vi "FindStartEndPointsRRT.vi"(8 "Goal":dbl[](array[numeric]), 9 "Initial State":dbl[](array[numeric]), 10 "Collision Points":dbl[][](array[numeric])) -> (1 "End Point RRT":dbl[](array[numeric]), 2 "Start Point RRT":dbl[](array[numeric]))   [LabVIEW 2017]
uses:
  <vilib>/Analysis/_algsub.llb/Real Vector Norm.vi
  <vilib>/Analysis/NI_AALPro.lvlib
panel:
  in  "tamanho minimo":dbl=200.0 format="%#_13g"
  out "Start Point RRT \na ser validado":dbl[](array[numeric])
  out "End Point RRT\na ser validado":dbl[](array[numeric])
  in  "threshold":dbl=400.0 format="%#_13g"
  out "Nearest Collision Point":dbl[](array[numeric])
  out "Furthest Collision Point":dbl[](array[numeric])
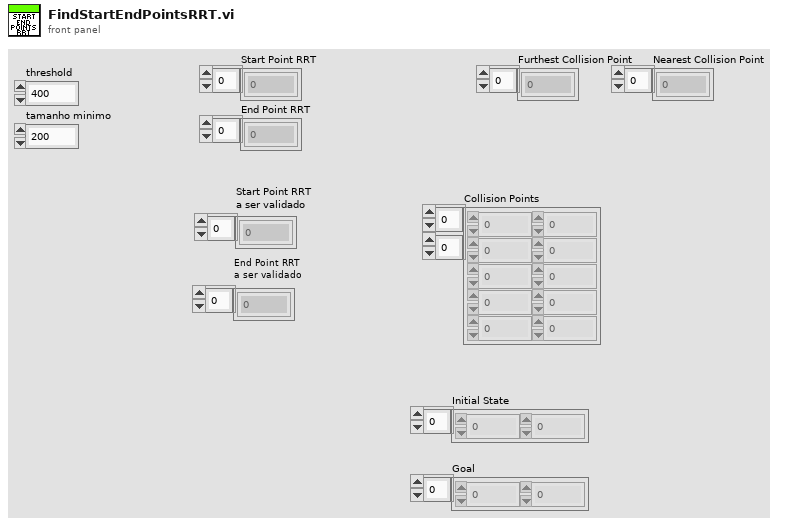
[diagram p1: front panel]
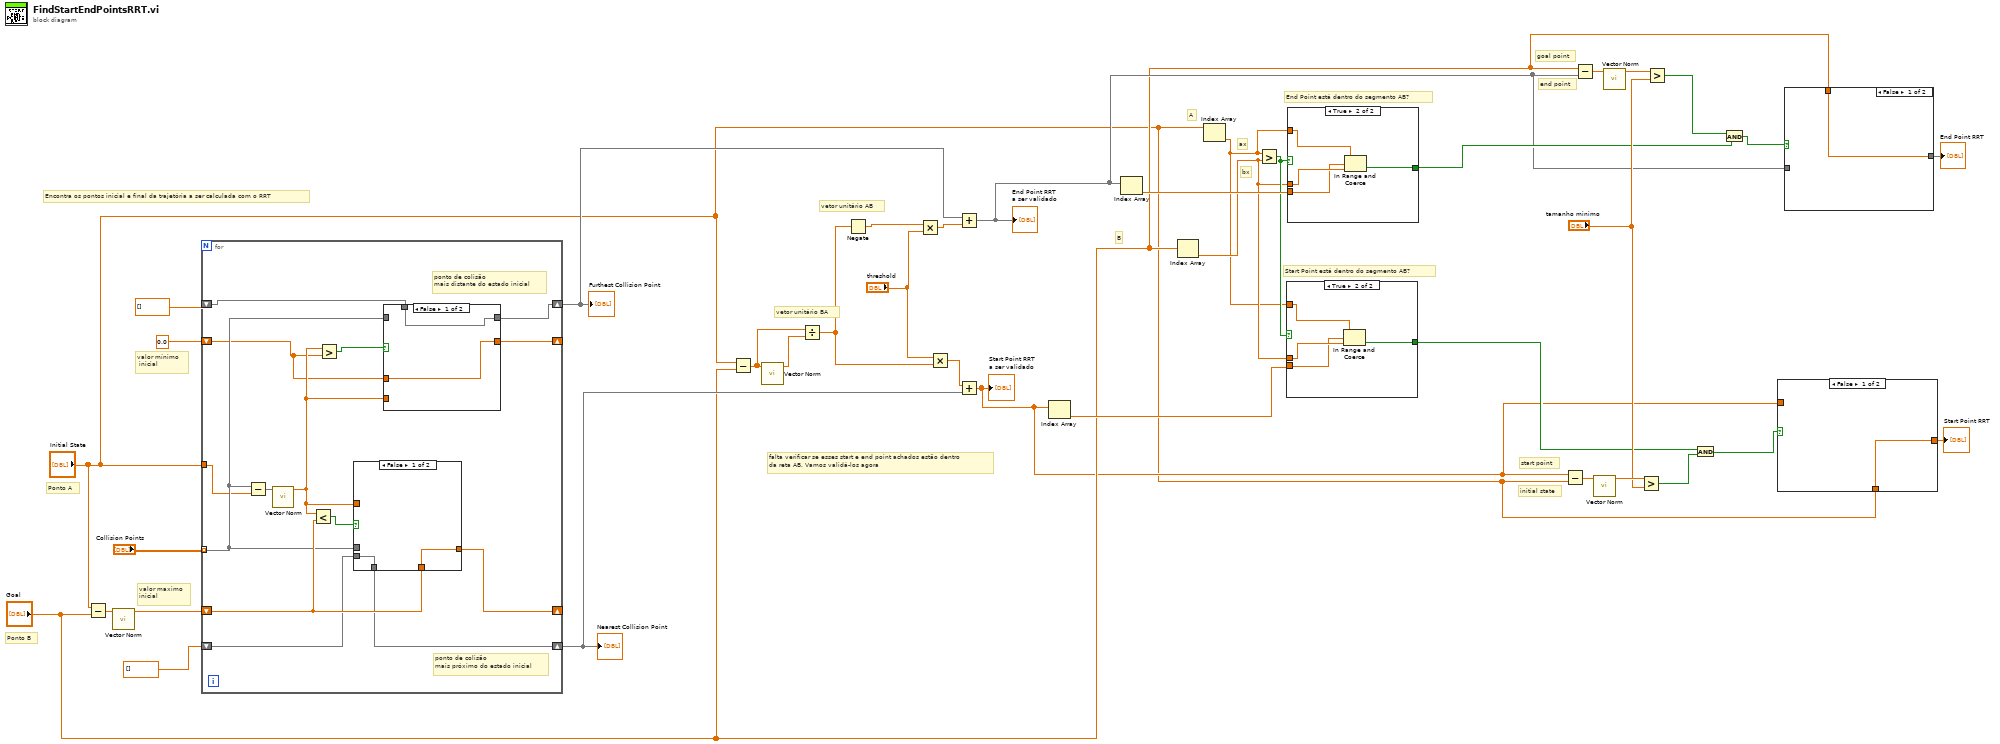
[diagram p0: block diagram]
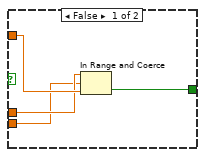
[diagram p4: hidden frame]
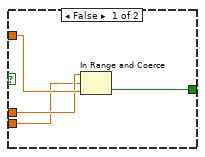
[diagram p5: hidden frame]
diagram:
  # "Encontra os pontos inicial e final da trajetória a ser calculada com o RRT"
  # "end point"
  # "goal point"
  # "initial state"
  # "start point"
  # "Start Point está dentro do segmento AB?"
  # "End Point está dentro do segmento AB?"
  # "bx"
  # "ax"
  # "B"
  # "A"
  # "falta verificar se esses start e end point achados estão dentro \nda reta AB. Vamos validá-los agora"
  # "vetor unitário AB"
  # "vetor unitário BA"
  # "valor mínimo\n inicial"
  # "valor maximo\ninicial"
  # "Ponto B"
  # "Ponto A"
  n1 = Subtract(x="Initial State", y="Goal") -> (x-y=w36:dbl[])
  n2 = call-poly <vilib>:"Vector Norm.vi"("Input Vector"=w36) -> ("norm"=w35:dbl)  [unwired: 9 in, 1 out]
  n3 = for {
    tunnel: "Collision Points" -> [w42] mode=indexing
    tunnel: "Initial State" -> [w38]
    shift-right: [w43] -> _
    shift-left: 0.0 -> [w40]
    shift-right: [w48] -> _
    shift-left: w35 -> [w49]
    shift-right: [w47] -> w23
    shift-left: dbl[] [] ("Goal 2") -> [w46]
    shift-right: [w41] -> w27
    shift-left: dbl[] [] ("Goal 2") -> [w39]
    # "ponto de colisão \nmais distante do estado inicial"
    # "ponto de colisão \nmais próximo do estado inicial"
    n4 = Subtract(x=w42, y=w38) -> (x-y=w51:dbl[])
    n5 = call-poly <vilib>:"Vector Norm.vi"("Input Vector"=w51) -> ("norm"=w44:dbl)  [unwired: 9 in, 1 out]
    n6 = Less?(x=w44, y=w49) -> (x < y?=w50:bool)
    n7 = Greater?(x=w44, y=w40) -> (0:w45:bool)
    n8 = case shown="False" w50 {
      tunnel: [w57 w59] -> w48
      tunnel: w44 -> [_ w59]
      tunnel: w49 -> [w57 _]
      tunnel: w42 -> [_ w58]
      tunnel: [w56 w58] -> w47
      tunnel: w46 -> [w56 _]
      frame False {
      }
      frame True {
      }
    }
    n9 = case shown="False" w45 {
      tunnel: w44 -> [_ w55]
      tunnel: [w53 w55] -> w43
      tunnel: w42 -> [_ w54]
      tunnel: [w52 w54] -> w41
      tunnel: w40 -> [w53 _]
      tunnel: w39 -> [w52 _]
      frame False {
      }
      frame True {
      }
    }
  }
  "Furthest Collision Point" <- w27
  "Nearest Collision Point" <- w23
  n10 = Subtract(x="Initial State", y="Goal") -> (x-y=w31:dbl[])
  n11 = call-poly <vilib>:"Vector Norm.vi"("Input Vector"=w31) -> ("norm"=w30:dbl)  [unwired: 9 in, 1 out]
  n12 = Divide(x=w31, y=w30) -> (x/y=w25:dbl[])
  n13 = Negate(x=w25) -> (-x=w29:dbl[])
  n14 = Multiply(x=w29, y="threshold") -> (x*y=w28:dbl[])
  n15 = Multiply(x="threshold", y=w25) -> (x*y=w24:dbl[])
  n16 = Add(x=w27, y=w28) -> (x+y=w7:dbl[])
  "End Point RRT\na ser validado" <- w7
  n17 = Add(x=w24, y=w23) -> (x+y=w4:dbl[])
  "Start Point RRT \na ser validado" <- w4
  n18 = Index Array(array=w4) -> (element=w20:dbl)  [unwired: 1 in]
  n19 = Index Array(array=w7) -> (element=w22:dbl)  [unwired: 1 in]
  n20 = Index Array(array="Goal") -> (element=w19:dbl)  [unwired: 1 in]
  n21 = Index Array(array="Initial State") -> (element=w18:dbl)  [unwired: 1 in]
  n22 = Greater?(x=w18, y=w19) -> (0:w21:bool)
  n23 = case shown="True" w21 {
    tunnel: w18 -> [w63 w67]
    tunnel: w19 -> [w62 w66]
    tunnel: w20 -> [w61 w65]
    tunnel: [w60 w64] -> w10
    frame False {
      n24 = In Range and Coerce(upper limit=w62, x=w61, lower limit=w63) -> (In Range?=w60:bool)  [unwired: 1 out]
    }
    frame True {
      n25 = In Range and Coerce(upper limit=w67, x=w65, lower limit=w66) -> (In Range?=w64:bool)  [unwired: 1 out]
    }
  }
  n26 = case shown="True" w21 {
    tunnel: w18 -> [w71 w75]
    tunnel: w19 -> [w70 w74]
    tunnel: w22 -> [w69 w73]
    tunnel: [w68 w72] -> w12
    frame False {
      n27 = In Range and Coerce(upper limit=w70, x=w69, lower limit=w71) -> (In Range?=w68:bool)  [unwired: 1 out]
    }
    frame True {
      n28 = In Range and Coerce(upper limit=w75, x=w73, lower limit=w74) -> (In Range?=w72:bool)  [unwired: 1 out]
    }
  }
  n29 = Subtract(x=w4, y="Initial State") -> (x-y=w17:dbl[])
  n30 = Subtract(x="Goal", y=w7) -> (x-y=w16:dbl[])
  n31 = call-poly <vilib>:"Vector Norm.vi"("Input Vector"=w17) -> ("norm"=w14:dbl)  [unwired: 9 in, 1 out]
  n32 = call-poly <vilib>:"Vector Norm.vi"("Input Vector"=w16) -> ("norm"=w15:dbl)  [unwired: 9 in, 1 out]
  n33 = Greater?(x=w14, y="tamanho minimo") -> (0:w9:bool)
  n34 = Greater?(x=w15, y="tamanho minimo") -> (0:w11:bool)
  n35 = And(x=w10, y=w9) -> (x .and. y?=w5:bool)
  n36 = And(x=w11, y=w12) -> (x .and. y?=w8:bool)
  n37 = case shown="False" w5 {
    tunnel: [w76 w77] -> w2
    tunnel: w4 -> [_ w77]
    tunnel: "Initial State" -> [w76 _]
    frame False {
    }
    frame True {
    }
  }
  "Start Point RRT" <- w2
  n38 = case shown="False" w8 {
    tunnel: w7 -> [_ w79]
    tunnel: [w78 w79] -> w1
    tunnel: "Goal" -> [w78 _]
    frame False {
    }
    frame True {
    }
  }
  "End Point RRT" <- w1
